vi "6229 Case Selection_Rev1.vi"(1 "Input Array":dbl[](array[numeric])) -> (0 "DAQ Channel Case":dbl)   [LabVIEW 2013]
uses:
  Instance          12 32Saved   6229 Case Selection_Rev1 .vi
  Instance          14 32Saved   6229 Case Selection_Rev1 .vi
  Instance          15 32Saved   6229 Case Selection_Rev1 .vi
  Instance          13 32Saved   6229 Case Selection_Rev1 .vi
  Instance           7 32Saved   6229 Case Selection_Rev1 .vi
  Instance           6 32Saved   6229 Case Selection_Rev1 .vi
  Instance           5 32Saved   6229 Case Selection_Rev1 .vi
  Instance           4 32Saved   6229 Case Selection_Rev1 .vi
  Instance           3 32Saved   6229 Case Selection_Rev1 .vi
  Instance           2 32Saved   6229 Case Selection_Rev1 .vi
  Instance           8 32Saved   6229 Case Selection_Rev1 .vi
  Instance           9 32Saved   6229 Case Selection_Rev1 .vi
  Instance          10 32Saved   6229 Case Selection_Rev1 .vi
  Instance          11 32Saved   6229 Case Selection_Rev1 .vi
  Instance           1 32Saved   6229 Case Selection_Rev1 .vi
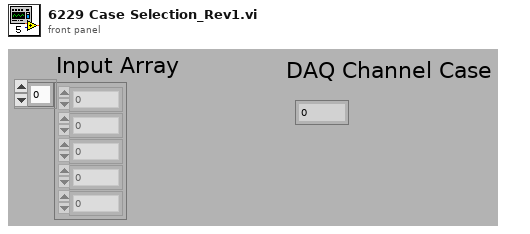
[diagram p1: front panel]
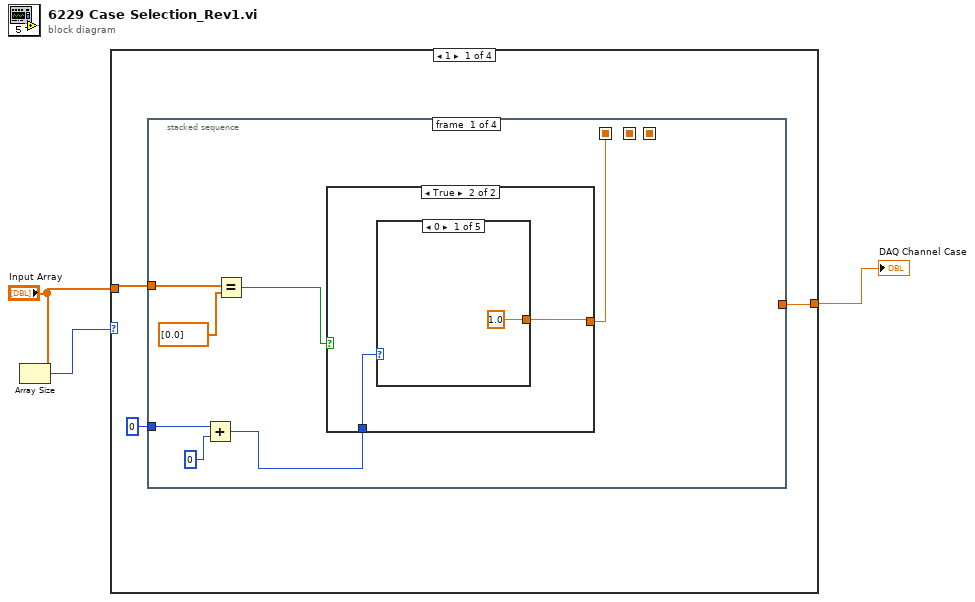
[diagram p0: block diagram]
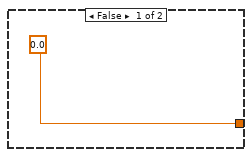
[diagram p2: hidden frame]
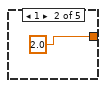
[diagram p3: hidden frame]
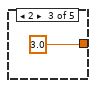
[diagram p4: hidden frame]
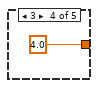
[diagram p5: hidden frame]
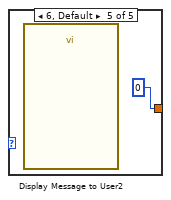
[diagram p6: hidden frame]
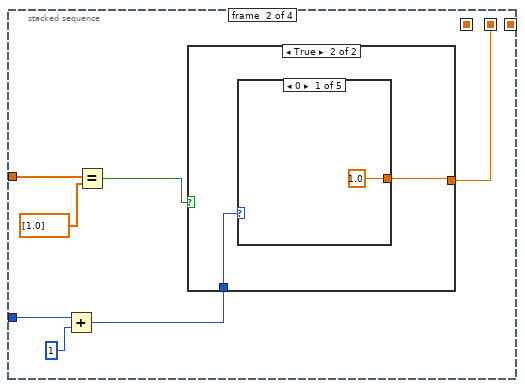
[diagram p7: hidden frame]
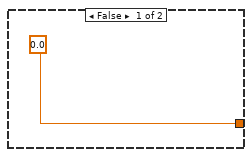
[diagram p8: hidden frame]
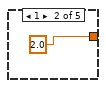
[diagram p9: hidden frame]
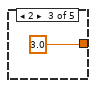
[diagram p10: hidden frame]
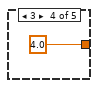
[diagram p11: hidden frame]
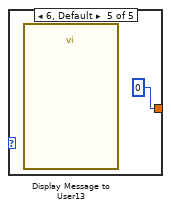
[diagram p12: hidden frame]
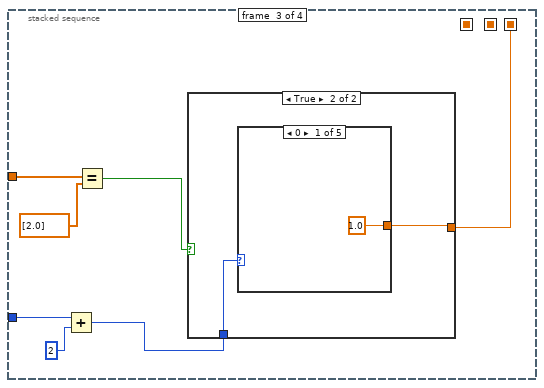
[diagram p13: hidden frame]
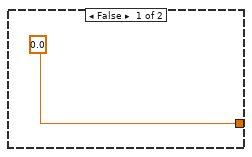
[diagram p14: hidden frame]
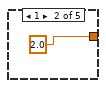
[diagram p15: hidden frame]
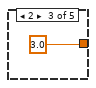
[diagram p16: hidden frame]
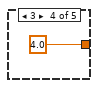
[diagram p17: hidden frame]
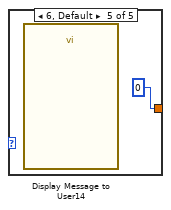
[diagram p18: hidden frame]
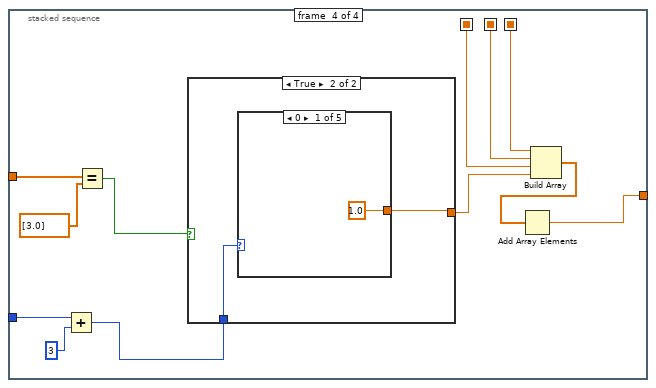
[diagram p19: hidden frame]
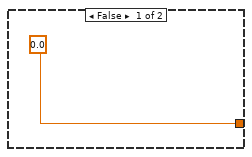
[diagram p20: hidden frame]
diagram:
  n1 = Array Size(array="Input Array") -> (size(s)=w3:i32)
  n2 = case shown="1" w3 {
    tunnel: "Input Array" -> [w6 w72 w185 w253]
    tunnel: [w4 w73 w184 w252] -> w1
    frame 1 {
      n3 = stacked-sequence {
        seq-local: [w7 _ _ _] -> [_ _ _ w55]
        seq-local: [_ w22 _ _] -> [_ _ _ w56]
        seq-local: [_ _ w39 _] -> [_ _ _ w57]
        tunnel: w6 -> [w13 w28 w43 w63]
        tunnel: 0 -> [w10 w25 w40 w60]
        tunnel: [_ _ _ w52] -> w4
        frame #0 {
          n4 = Add(x=w10, y=0) -> (x+y=w9:i32)
          n5 = Equal?(x=w13, y=dbl[] [0.0]) -> (x = y?=w8:bool)
          n6 = case shown="True" w8 {
            tunnel: [0.0 w16] -> w7
            tunnel: w9 -> [_ w15]
            frame False {
            }
            frame True {
              n7 = case shown="0" w15 {
                tunnel: [1.0 2.0 3.0 4.0 0] -> w16
                frame 0 {
                }
                frame 1 {
                }
                frame 2 {
                }
                frame 3 {
                }
                frame 6, Default {
                  n8 = call "Display Message to User2"() -> ()  [unwired: 10 in, 2 out]
                }
              }
            }
          }
        }
        frame #1 {
          n9 = Add(x=w25, y=1) -> (x+y=w23:i32)
          n10 = Equal?(x=w28, y=dbl[] [1.0]) -> (x = y?=w24:bool)
          n11 = case shown="True" w24 {
            tunnel: [0.0 w31] -> w22
            tunnel: w23 -> [_ w30]
            frame False {
            }
            frame True {
              n12 = case shown="0" w30 {
                tunnel: [1.0 2.0 3.0 4.0 0] -> w31
                frame 0 {
                }
                frame 1 {
                }
                frame 2 {
                }
                frame 3 {
                }
                frame 6, Default {
                  n13 = call "Display Message to User13"() -> ()  [unwired: 10 in, 2 out]
                }
              }
            }
          }
        }
        frame #2 {
          n14 = Add(x=w40, y=2) -> (x+y=w37:i32)
          n15 = Equal?(x=w43, y=dbl[] [2.0]) -> (x = y?=w38:bool)
          n16 = case shown="True" w38 {
            tunnel: [0.0 w46] -> w39
            tunnel: w37 -> [_ w45]
            frame False {
            }
            frame True {
              n17 = case shown="0" w45 {
                tunnel: [1.0 2.0 3.0 4.0 0] -> w46
                frame 0 {
                }
                frame 1 {
                }
                frame 2 {
                }
                frame 3 {
                }
                frame 6, Default {
                  n18 = call "Display Message to User14"() -> ()  [unwired: 10 in, 2 out]
                }
              }
            }
          }
        }
        frame #3 {
          n19 = Add(x=w60, y=3) -> (x+y=w59:i32)
          n20 = Equal?(x=w63, y=dbl[] [3.0]) -> (x = y?=w58:bool)
          n21 = case shown="True" w58 {
            tunnel: [0.0 w66] -> w54
            tunnel: w59 -> [_ w65]
            frame False {
            }
            frame True {
              n22 = case shown="0" w65 {
                tunnel: [1.0 2.0 3.0 4.0 0] -> w66
                frame 0 {
                }
                frame 1 {
                }
                frame 2 {
                }
                frame 3 {
                }
                frame 6, Default {
                  n23 = call "Display Message to User17"() -> ()  [unwired: 10 in, 2 out]
                }
              }
            }
          }
          n24 = Build Array(w57, w56, w55, w54) -> (w53:dbl[])
          n25 = Add Array Elements(numeric array=w53) -> (sum=w52:dbl)
        }
      }
    }
    frame 2 {
      n26 = stacked-sequence {
        seq-local: [w75 _ _ _ _ _] -> [_ _ _ _ _ w163]
        seq-local: [_ w92 _ _ _ _] -> [_ _ _ _ _ w164]
        seq-local: [_ _ w109 _ _ _] -> [_ _ _ _ _ w165]
        seq-local: [_ _ _ w126 _ _] -> [_ _ _ _ _ w166]
        seq-local: [_ _ _ _ w143 _] -> [_ _ _ _ _ w167]
        tunnel: w72 -> [w81 w98 w115 w132 w149 w173]
        tunnel: 0 -> [w78 w95 w112 w129 w146 w170]
        tunnel: [_ _ _ _ _ w160] -> w73
        frame #0 {
          n27 = Add(x=w78, y=0) -> (x+y=w77:i32)
          n28 = Equal?(x=w81, y=dbl[] [0.0, 1.0]) -> (x = y?=w76:bool)
          n29 = case shown="True" w76 {
            tunnel: [0.0 w84] -> w75
            tunnel: w77 -> [_ w83]
            frame False {
            }
            frame True {
              n30 = case shown="0" w83 {
                tunnel: [5.0 6.0 7.0 8.0 9.0 10.0 0] -> w84
                frame 0 {
                }
                frame 1 {
                }
                frame 2 {
                }
                frame 3 {
                }
                frame 4 {
                }
                frame 5 {
                }
                frame 6, Default {
                  n31 = call "Display Message to User3"() -> ()  [unwired: 10 in, 2 out]
                }
              }
            }
          }
        }
        frame #1 {
          n32 = Add(x=w95, y=1) -> (x+y=w94:i32)
          n33 = Equal?(x=w98, y=dbl[] [0.0, 2.0]) -> (x = y?=w93:bool)
          n34 = case shown="True" w93 {
            tunnel: [0.0 w101] -> w92
            tunnel: w94 -> [_ w100]
            frame False {
            }
            frame True {
              n35 = case shown="1" w100 {
                tunnel: [5.0 6.0 7.0 8.0 9.0 10.0 0] -> w101
                frame 0 {
                }
                frame 1 {
                }
                frame 2 {
                }
                frame 3 {
                }
                frame 4 {
                }
                frame 5 {
                }
                frame 6, Default {
                  n36 = call "Display Message to User4"() -> ()  [unwired: 10 in, 2 out]
                }
              }
            }
          }
        }
        frame #2 {
          n37 = Add(x=w112, y=2) -> (x+y=w111:i32)
          n38 = Equal?(x=w115, y=dbl[] [0.0, 3.0]) -> (x = y?=w110:bool)
          n39 = case shown="True" w110 {
            tunnel: [0.0 w118] -> w109
            tunnel: w111 -> [_ w117]
            frame False {
            }
            frame True {
              n40 = case shown="2" w117 {
                tunnel: [5.0 6.0 7.0 8.0 9.0 10.0 0] -> w118
                frame 0 {
                }
                frame 1 {
                }
                frame 2 {
                }
                frame 3 {
                }
                frame 4 {
                }
                frame 5 {
                }
                frame 6, Default {
                  n41 = call "Display Message to User5"() -> ()  [unwired: 10 in, 2 out]
                }
              }
            }
          }
        }
        frame #3 {
          n42 = Add(x=w129, y=3) -> (x+y=w128:i32)
          n43 = Equal?(x=w132, y=dbl[] [1.0, 2.0]) -> (x = y?=w127:bool)
          n44 = case shown="True" w127 {
            tunnel: [0.0 w135] -> w126
            tunnel: w128 -> [_ w134]
            frame False {
            }
            frame True {
              n45 = case shown="3" w134 {
                tunnel: [5.0 6.0 7.0 8.0 9.0 10.0 0] -> w135
                frame 0 {
                }
                frame 1 {
                }
                frame 2 {
                }
                frame 3 {
                }
                frame 4 {
                }
                frame 5 {
                }
                frame 6, Default {
                  n46 = call "Display Message to User6"() -> ()  [unwired: 10 in, 2 out]
                }
              }
            }
          }
        }
        frame #4 {
          n47 = Add(x=w146, y=4) -> (x+y=w145:i32)
          n48 = Equal?(x=w149, y=dbl[] [1.0, 3.0]) -> (x = y?=w144:bool)
          n49 = case shown="True" w144 {
            tunnel: [0.0 w152] -> w143
            tunnel: w145 -> [_ w151]
            frame False {
            }
            frame True {
              n50 = case shown="4" w151 {
                tunnel: [5.0 6.0 7.0 8.0 9.0 10.0 0] -> w152
                frame 0 {
                }
                frame 1 {
                }
                frame 2 {
                }
                frame 3 {
                }
                frame 4 {
                }
                frame 5 {
                }
                frame 6, Default {
                  n51 = call "Display Message to User7"() -> ()  [unwired: 10 in, 2 out]
                }
              }
            }
          }
        }
        frame #5 {
          n52 = Add(x=w170, y=5) -> (x+y=w169:i32)
          n53 = Equal?(x=w173, y=dbl[] [2.0, 3.0]) -> (x = y?=w168:bool)
          n54 = case shown="True" w168 {
            tunnel: [0.0 w176] -> w162
            tunnel: w169 -> [_ w175]
            frame False {
            }
            frame True {
              n55 = case shown="5" w175 {
                tunnel: [5.0 6.0 7.0 8.0 9.0 10.0 0] -> w176
                frame 0 {
                }
                frame 1 {
                }
                frame 2 {
                }
                frame 3 {
                }
                frame 4 {
                }
                frame 5 {
                }
                frame 6, Default {
                  n56 = call "Display Message to User8"() -> ()  [unwired: 10 in, 2 out]
                }
              }
            }
          }
          n57 = Build Array(w167, w166, w165, w164, w163, w162) -> (w161:dbl[])
          n58 = Add Array Elements(numeric array=w161) -> (sum=w160:dbl)
        }
      }
    }
    frame 3 {
      n59 = stacked-sequence {
        seq-local: [w187 _ _ _] -> [_ _ _ w236]
        seq-local: [_ w202 _ _] -> [_ _ _ w237]
        seq-local: [_ _ w217 _] -> [_ _ _ w234]
        tunnel: w185 -> [w193 w208 w223 w243]
        tunnel: 0 -> [w190 w205 w220 w240]
        tunnel: [_ _ _ w232] -> w184
        frame #0 {
          n60 = Add(x=w190, y=0) -> (x+y=w189:i32)
          n61 = Equal?(x=w193, y=dbl[] [0.0, 1.0, 2.0]) -> (x = y?=w188:bool)
          n62 = case shown="True" w188 {
            tunnel: [0.0 w196] -> w187
            tunnel: w189 -> [_ w195]
            frame False {
            }
            frame True {
              n63 = case shown="0" w195 {
                tunnel: [11.0 12.0 13.0 14.0 0] -> w196
                frame 0 {
                }
                frame 1 {
                }
                frame 2 {
                }
                frame 3 {
                }
                frame 6, Default {
                  n64 = call "Display Message to User11"() -> ()  [unwired: 10 in, 2 out]
                }
              }
            }
          }
        }
        frame #1 {
          n65 = Add(x=w205, y=1) -> (x+y=w204:i32)
          n66 = Equal?(x=w208, y=dbl[] [0.0, 1.0, 3.0]) -> (x = y?=w203:bool)
          n67 = case shown="True" w203 {
            tunnel: [0.0 w211] -> w202
            tunnel: w204 -> [_ w210]
            frame False {
            }
            frame True {
              n68 = case shown="1" w210 {
                tunnel: [11.0 12.0 13.0 14.0 0] -> w211
                frame 0 {
                }
                frame 1 {
                }
                frame 2 {
                }
                frame 3 {
                }
                frame 6, Default {
                  n69 = call "Display Message to User9"() -> ()  [unwired: 10 in, 2 out]
                }
              }
            }
          }
        }
        frame #2 {
          n70 = Add(x=w220, y=2) -> (x+y=w219:i32)
          n71 = Equal?(x=w223, y=dbl[] [0.0, 2.0, 3.0]) -> (x = y?=w218:bool)
          n72 = case shown="True" w218 {
            tunnel: [0.0 w226] -> w217
            tunnel: w219 -> [_ w225]
            frame False {
            }
            frame True {
              n73 = case shown="2" w225 {
                tunnel: [11.0 12.0 13.0 14.0 0] -> w226
                frame 0 {
                }
                frame 1 {
                }
                frame 2 {
                }
                frame 3 {
                }
                frame 6, Default {
                  n74 = call "Display Message to User10"() -> ()  [unwired: 10 in, 2 out]
                }
              }
            }
          }
        }
        frame #3 {
          n75 = Add(x=w240, y=3) -> (x+y=w239:i32)
          n76 = Equal?(x=w243, y=dbl[] [1.0, 2.0, 3.0]) -> (x = y?=w238:bool)
          n77 = case shown="True" w238 {
            tunnel: [0.0 w246] -> w233
            tunnel: w239 -> [_ w245]
            frame False {
            }
            frame True {
              n78 = case shown="3" w245 {
                tunnel: [11.0 12.0 13.0 14.0 0.0] -> w246
                frame 0 {
                }
                frame 1 {
                }
                frame 2 {
                }
                frame 3 {
                }
                frame 4, Default {
                  n79 = call "Display Message to User12"() -> ()  [unwired: 10 in, 2 out]
                }
              }
            }
          }
          n80 = Build Array(w234, w237, w236, w233) -> (w235:dbl[])
          n81 = Add Array Elements(numeric array=w235) -> (sum=w232:dbl)
        }
      }
    }
    frame 4, Default {
      n82 = Equal?(x=w253, y=dbl[] [0.0, 1.0, 2.0, 3.0]) -> (x = y?=w254:bool)
      n83 = case shown="True" w254 {
        tunnel: [-1 15.0] -> w252
        frame False {
          n84 = call "Display Message to User"("Enable"=TRUE) -> ()  [unwired: 9 in, 2 out]
        }
        frame True {
        }
      }
    }
  }
  "DAQ Channel Case" <- w1
